vi "hours_to_mins.vi"(9 "minute(00-59)":i32, 11 "hour(00-23)":i32) -> (3 "hr+min":i32)   [LabVIEW 2011]
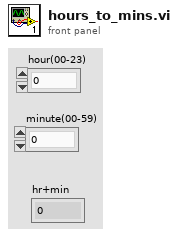
[diagram p1: front panel]
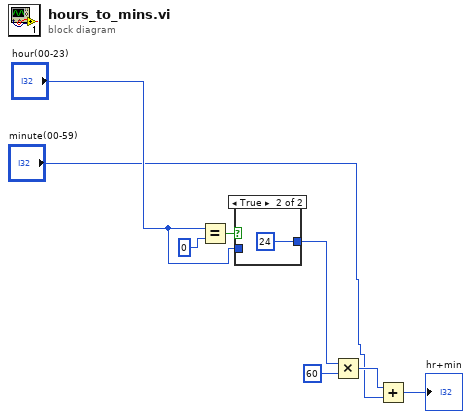
[diagram p0: block diagram]
diagram:
  n1 = Equal?(x="hour(00-23)", y=0) -> (x = y?=w5:bool)
  n2 = case shown="True" w5 {
    tunnel: [w9 24] -> w2
    tunnel: "hour(00-23)" -> [w9 _]
    frame False {
    }
    frame True {
    }
  }
  n3 = Multiply(x=w2, y=60) -> (x*y=w7:i32)
  n4 = Add(x=w7, y="minute(00-59)") -> (x+y=→"hr+min":i32)
